vi "Lab1.vi"() -> ()   [LabVIEW 2019]
doc: "Simulator of heater model with PI controller, filter and datalogging"
uses:
  <vilib>/OPCUA/controls/NodeId.ctl
  <vilib>/OPCUA/controls/Write Status.ctl
  <vilib>/Simulation/Scripting/Companion Diagram/SimConfigNode/SimParams.ctl
  <vilib>/Simulation/Scripting/Companion Diagram/SimConfigNode/_simSolvers.ctl
  <vilib>/Simulation/Implementation/Shared/SIMSCR Execution Mode.ctl
  <vilib>/Simulation/Param Hierarchy/Typedefs/SIMPH Param Control Actions.ctl
  <vilib>/Simulation/Implementation/Shared/NILVSim_ParamChanged.vi
  <vilib>/Simulation/Implementation/Shared/NILVSIM_BeginStep.vi
  <vilib>/Simulation/Implementation/Shared/NILVSim_Manager.vi
  <vilib>/Utility/error.llb/Clear Errors.vi
  <vilib>/Simulation/Implementation/Shared/NILVSim_FinalizeModel.vi
  <vilib>/Simulation/Implementation/Shared/SIM Unbundle Sim Info.vi
  <vilib>/Simulation/Implementation/Shared/NILVSim_Initialize.vi
  <vilib>/Simulation/Utility/Implementation/NILVSim Get Time and IsAcceptedStep.vi
  <vilib>/Simulation/Implementation/Shared/SIMSH Read Queue.vi
  <vilib>/Simulation/Implementation/Shared/NILVSim_GetModelError.vi
  <vilib>/Simulation/Implementation/Shared/SIM Bundle Sim Info.vi
  <vilib>/OPCUA/client/Multiple Write Double.vi
  <vilib>/Simulation/Implementation/XNodeFramework/SimXNode/SimX.xnode
  Air Heater Black Box Model.vi
  <vilib>/Simulation/Scripting/Companion Diagram/SimConfigNode/SimDog.xnode
  Sim with delay.vi
  <vilib>/OPCUA/NI OPC UA Client.lvlib
  <vilib>/Simulation/Implementation/Shared/NI_SIM_Implementation.lvlib
panel:
  in  "stop":bool=TRUE
  out "Waveform Chart 2":dbl(graph)=4.205713068274385
  in  "Tab Control":T1(tab)=enum."OPC-UA"
  in  "Temperature setpoint":dbl(knob)=24.003099081961754 scale=20.0..50.0
  in  "auto_man":bool=TRUE
  in  "man_output u [V]":dbl
  out "u":dbl=4.205713068274385
  in  "Ti":dbl=12.0 format="%.3f"
  in  "Kp":dbl=1.2 format="%.3f"
  out "y":dbl=21.680348521334466
  in  "Process Mode":string(combo)="Black Box"
  in  "Kh":dbl=3.5
  in  "theta_t":dbl=22.0
  in  "theta_d":dbl=2.0
  in  "T_env":dbl=21.0
  in  "Server Endpoint URL":string="opc.tcp://DESKTOP-2K1CGSL:49580"
  in  "Node Id":string="ns=2;s=Process Data.Temperature"
  out "Waveform Chart":T2(graph)={"Temperature setpoint"=24.003099081961754, "T_env"=21.680348521334466, "T_out"=0.0}
  # "Auto"
  # "Man"
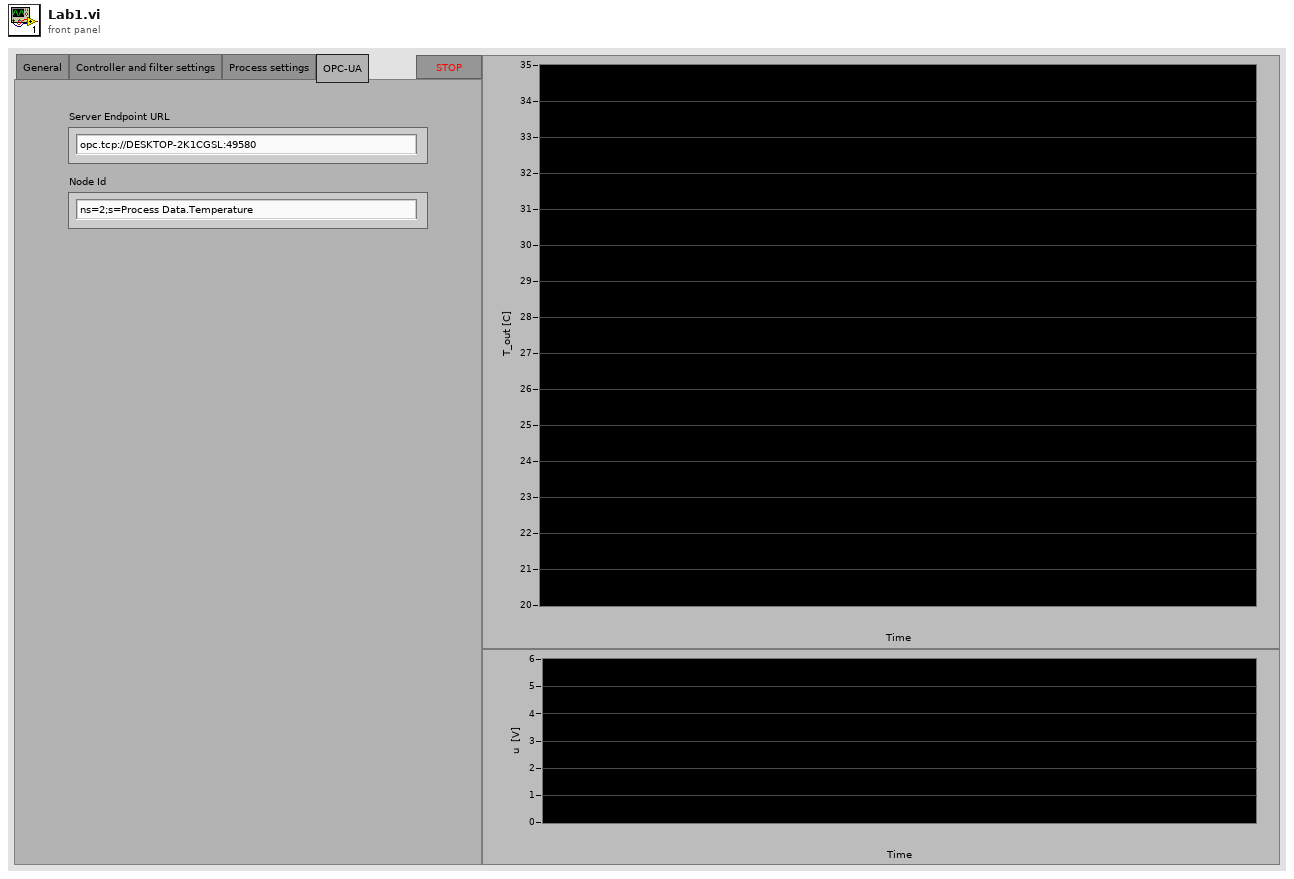
[diagram p1: front panel]
types:
  T1 = enum32{"General", "Controller and filter settings", "Process settings", "OPC-UA"}
  T2 = cluster{"Temperature setpoint":dbl, "T_env":dbl, "T_out":dbl}
  T3 = cluster{"Temperature setpoint":dbl, "T_env":dbl, "T_out":dbl}[]
  T4 = cluster{"message mode":enum16{"None", "Sign", "Sign and Encrypt"}, "security":enum16{"Basic256", "Basic128Rsa15"}}
  T5 = enum16{"Simulate to Completion", "Single Time-Step Simulation (Fixed Step Only)"}
  T6 = typedef "SIMSCR Execution Mode.ctl" = enum16{"Simulate to Completion", "Single Time-Step Simulation (Fixed Step Only)"}
  T7 = typedef "SIMPH Param Control Actions.ctl" = enum16{"get params", "set params"}
  T8 = cluster{"SIMSH Sim Time":dbl, "Select":cluster{"s? t:f":dbl}, "Linear Scaling with Points.vi":cluster{"y":dbl}, "Summation 3":cluster{"Result":dbl}, "Square Root":cluster{"sqrt(x)":dbl}, "Gaussian White Noise PtByPt.vi":cluster{"Gaussian white noise":dbl}, "Integrator":cluster{"output":dbl}, "Multiplication":cluster{"Result":dbl}, "Summation":cluster{"Result":dbl}, "Multiplication 2":cluster{"Result":dbl}, "Transport Delay":cluster{"output":dbl}, "Summation 2":cluster{"Result":dbl}}
  T9 = typedef "SimParams.ctl" = cluster{"Initial Time (s)":dbl, "Final Time (s)":dbl, "Step Size (s)":dbl, "ODE Solver":T10, "Minimum Step Size (s)":dbl, "Maximum Step Size (s)":dbl, "Relative Tolerance":dbl, "Absolute Tolerance":dbl, "Software Timing":bool, "Initial Step Size (s)":dbl, "Automatic Fixed Step Size?":bool, "Automatic Discrete Step Size?":bool, "Discrete Step Size (s)":dbl, "Calculate using Time Step":bool, "Solver Wired?":bool, "Prev.Frm.Expected End":u64, "Prev.Frm.Actual End":u64, "Prev.Frm.Finished Late?":bool, "Prev.Iter.Expected End":u64, "Prev.Iter.Actual End":u64, "Prev.Iter.Finished Late?":bool, "Expected Iteration Start":u64, "Actual Iteration Start":u64, "Expected Frame Start":u64, "Actual Frame Start":u64, "Source Name":string, "Name":string, "Period":i64, "Deadline":i64, "Offset":i64, "Start":i64, "Priority":i32, "Timeout":i32, "Processor":i32, "Mode":enum32{"No Change", "Process missed periods, maintain original phase", "Discard missed periods, maintain original phase", "Process missed periods, ignore original phase", "Discard missed periods, ignore original phase"}, "Wakeup reason":enum32{"Normal", "Aborted", "Asynchronous wakeup", "Timing source error", "Timed loop error", "Timeout"}, "Error":errorcluster, "Source Type":string, "Secondary Source Type":string, "Global End Time":u64, "Global Start Time":u64, "Full Solver Reset":bool, "Execution Mode":T6, "Nan/Inf Check":bool, "Custom Solver Library":string, "Solver Is Variable":bool, "custom solver name":string, "Signal Collection Decimation":u32}
  T10 = typedef "_simSolvers.ctl" = enum16{"Runge-Kutta 1 (Euler)", "Runge-Kutta 2", "Runge-Kutta 3", "Runge-Kutta 4", "Runge-Kutta 23 (variable)", "Runge-Kutta 45 (variable)", "BDF (variable)", "Adams-Moulton (variable)", "Rosenbrock (variable)", "Discrete States Only", "SDIRK 4 (variable)", "Radau 5 (variable)", "Radau 9 (variable)", "Radau 13 (variable)", "Radau [Variable Order] (variable)", "Gear's Method (variable)", "Linearizer", "State Query", "Trim Eval", "Custom Solver"}
  T11 = cluster{"SIMSH Sim Time":dbl, "upper limit":dbl, "Integrator":cluster{"output":dbl}, "Multiplication 2":cluster{"Result":dbl}, "Summation 2":cluster{"Result":dbl}, "Summation":cluster{"Result":dbl}, "Multiplication":cluster{"Result":dbl}, "Transport Delay":cluster{"output":dbl}}
  T12 = typedef "OPC UA Client Refnum.ctl" = refnum<k21>
  T13 = typedef "NodeId.ctl" = string
  T14 = typedef "Write Status.ctl" = u32
  T15 = cluster{"node ID":T13, "value":dbl, "timestamp (current time)":timestamp, "node status":T14}
  T16 = cluster{"Temperature setpoint":dbl, "Filter Output":dbl, "Tf [s]":dbl}
  T17 = cluster{"Temperature setpoint":dbl, "Filter Output":dbl, "T_out":dbl}
  T18 = cluster{"node ID":T13, "value":dbl, "timestamp (current time)":timestamp, "node status":T14}[]
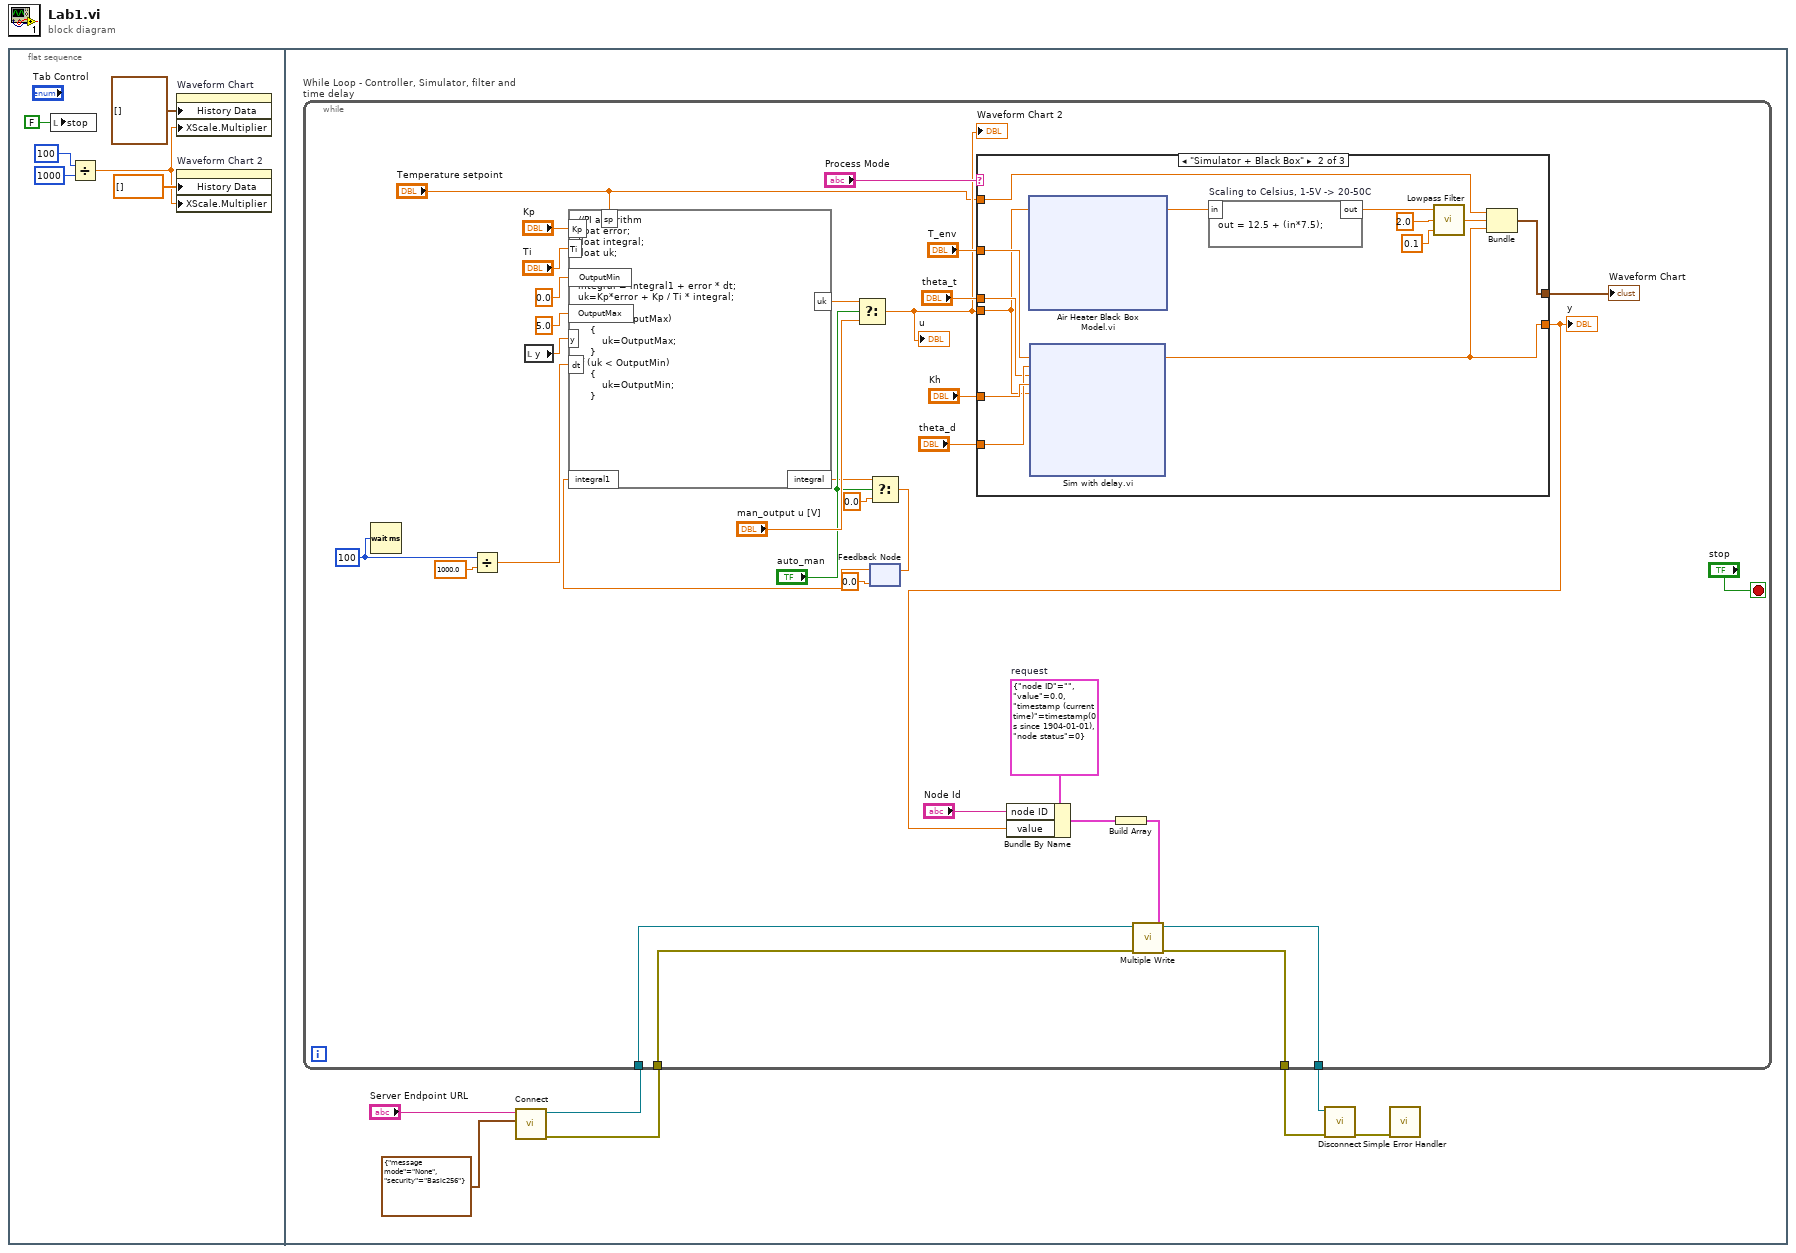
[diagram p0: block diagram]
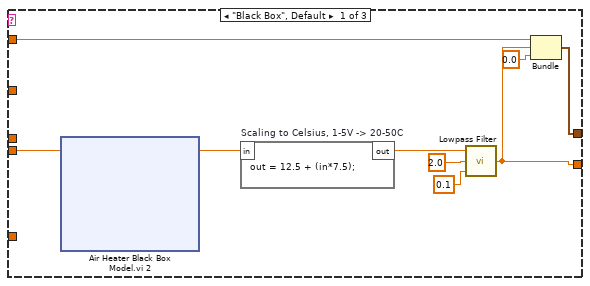
[diagram p2: hidden frame]
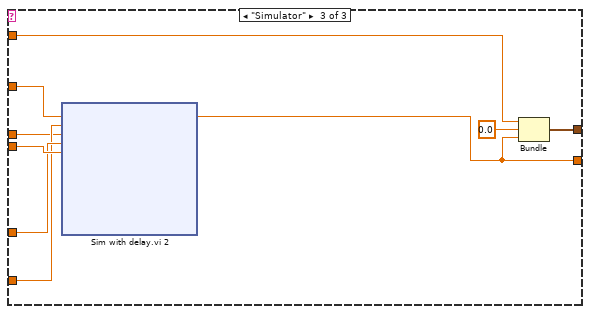
[diagram p3: hidden frame]
diagram:
  n1 = flat-sequence {
    frame #0 {
      n2 = local write "stop"(FALSE ("stop")) -> ()
      n3 = Divide(x=u32 100 ("milliseconds to wait"), y=u32 1000 ("x")) -> (x/y=w3:dbl)
      n4 = property on="Waveform Chart" class="WFChart (strict)"("History Data"=T3 [], "XScale.Multiplier"=w3) -> ()  [unwired: 2 in, 2 out]
      n5 = property on="Waveform Chart 2" class="WFChart (strict)"("History Data"=dbl[] [], "XScale.Multiplier"=w3) -> ()  [unwired: 2 in, 2 out]
    }
    frame #1 {
      n6 = call <vilib>:"Connect.vi"("security policy"=T4 {"message mode"=enum."None", "security"=enum."Basic256"}, "server endpoint URL"="Server Endpoint URL") -> ("error out"=w11:errorcluster, "OPC UA client refnum out"=w10:T12)  [unwired: 7 in, 1 out]
      n7 = while "While Loop - Controller, Simulator, filter and time delay" {
        tunnel: w11 -> [w15]
        tunnel: w10 -> [w16]
        tunnel: [w18] -> w8
        tunnel: [w17] -> w7
        stop <- "stop" stop-if-true
        w20 = T15 {"node ID"="", "value"=0.0, "timestamp (current time)"=timestamp(0 s since 1904-01-01), "node status"=0}  # request
        w36 = u32 100 ("milliseconds to wait")
        n8 = Wait (ms)(milliseconds to wait=w36) -> ()  [unwired: 1 out]
        n9 = Divide(x=w36, y=1000.0) -> (x/y=w35:dbl)
        n10 = local read "y"() -> (w38:dbl)
        n11 = feedback #1(0.0) -> (w32:dbl)
        n12 = formula code="//PI algorithm\nfloat error;\nfloat integral;\nfloat uk;\n\nerror=sp-y;\nintegral = integral1 + error * dt;\nuk=Kp*error + Kp / Ti * integral;\n\nif (uk > OutputMax)\n    {\n        uk=OutputMax;\n    }\nif (uk < OutputMin)\n    {\n        uk=OutputMin;\n    }"("Kp"="Kp", "Ti"="Ti", "OutputMin"=0.0 ("input variable"), "OutputMax"=5.0 ("input variable"), "y"=w38, "dt"=w35, "integral1"=w32, "sp"="Temperature setpoint") -> ("uk"=w29:dbl, "integral"=w26:dbl)
        n13 = Select(t=w29, s="auto_man", f="man_output u [V]") -> (s? t:f=w30:dbl)
        "Waveform Chart 2" <- w30
        "u" <- w30
        n14 = Select(t=w26, s="auto_man", f=0.0) -> (s? t:f=w25:dbl)
        n15 = feedback-in #1(w25) -> ()
        n16 = case shown="\"Simulator + Black Box\"" "Process Mode" {
          tunnel: [w49 w313 w832] -> w14
          tunnel: w30 -> [w53 w303 w831]
          tunnel: [w51 w308 w834] -> w46
          tunnel: "Kh" -> [_ w307 w830]
          tunnel: "T_env" -> [_ w306 w828]
          tunnel: "theta_d" -> [_ w305 w829]
          tunnel: "theta_t" -> [_ w304 w827]
          tunnel: "Temperature setpoint" -> [w48 w302 w826]
          frame "Black Box", Default {
            n17 = xnode "Air Heater Black Box Model.vi 2"("Control Signal [0-5V]"=w53) -> ("Tout [1-5V]"=w52:dbl)  [unwired: 2 in, 1 out]
            n18 = formula code="out = 12.5 + (in*7.5);" "Scaling to Celsius, 1-5V -> 20-50C"("in"=w52) -> ("out"=w56:dbl)
            n19 = call "Lowpass Filter.vi"("Ts [s]"=0.1, "Tf [s]"=2.0, "Filter Input"=w56) -> ("Filter Output"=w49:dbl)
            n20 = Bundle("Temperature setpoint"=w48, "Filter Output"=w49, "Tf [s]"=0.0) -> (w51:T16)  [unwired: 1 in]
          }
          frame "Simulator + Black Box" {
            n21 = xnode "Air Heater Black Box Model.vi"("Control Signal [0-5V]"=w303) -> ("Tout [1-5V]"=w314:dbl)  [unwired: 2 in, 1 out]
            n22 = xnode "Sim with delay.vi"("T_env"=w306, "theta_d"=w305, "theta_t"=w304, "Kh"=w307, "u"=w303) -> ("T_out"=w313:dbl)  [unwired: 2 in, 7 out]
            n23 = formula code="out = 12.5 + (in*7.5);" "Scaling to Celsius, 1-5V -> 20-50C"("in"=w314) -> ("out"=w312:dbl)
            n24 = call "Lowpass Filter.vi"("Ts [s]"=0.1, "Tf [s]"=2.0, "Filter Input"=w312) -> ("Filter Output"=w309:dbl)
            n25 = Bundle("Temperature setpoint"=w302, "Filter Output"=w309, "T_out"=w313) -> (w308:T17)  [unwired: 1 in]
          }
          frame "Simulator" {
            n26 = xnode "Sim with delay.vi 2"("T_env"=w828, "theta_d"=w829, "theta_t"=w827, "Kh"=w830, "u"=w831) -> ("T_out"=w832:dbl)  [unwired: 2 in, 7 out]
            n27 = Bundle("Temperature setpoint"=w826, "T_env"=0.0, "T_out"=w832) -> (w834:T2)  [unwired: 1 in]
          }
        }
        "Waveform Chart" <- w46
        "y" <- w14
        n28 = Bundle By Name "Bundle By Name"(cluster=w20, "node ID"="Node Id", "value"=w14) -> (w21:T15)
        n29 = Build Array(w21) -> (w19:T18)
        n30 = call-poly <vilib>:"Multiple Write.vi"("error in (no error)"=w15, "requests"=w19, "OPC UA client refnum in"=w16) -> ("error out"=w17:errorcluster, "OPC UA client refnum out"=w18:T12)  [unwired: 5 in, 2 out]
      }
      n31 = call <vilib>:"Disconnect.vi"("error in (no error)"=w7, "OPC UA client refnum in"=w8) -> ("error out"=w9:errorcluster)  [unwired: 9 in]
      n32 = call <vilib>:"Simple Error Handler.vi"("error in (no error)"=w9) -> ()  [unwired: 4 in, 5 out]
    }
  }
